vi "Day 2.vi"() -> ()   [LabVIEW 2018]
panel:
  in  "Boolean 2":bool
  in  "Boolean":bool
  in  "Ring":u16(ring)
  in  "Enum":enum16{""}(ring)
  out "x*y":i32
  out "Numeric 2":i32
  out "output cluster 2":cluster{"Numeric 9":dbl, "String":string}
  in  "Cluster 2":cluster{"Numeric 9":dbl, "String":string}
  out "output cluster":T1
  in  "Cluster":T1
  out "x+y":dbl[](array[numeric])
  in  "Array 3":dbl[](array[numeric])
  out "subarray":dbl[][](array[numeric])
  out "min index(es)":i32[](array[numeric])
  out "min value":dbl
  out "max value 2":dbl
  out "max index(es)":i32[](array[numeric])
  in  "max value":dbl
  out "element":dbl
  out "array w/ subset deleted":dbl[](array[numeric])
  out "deleted portion":dbl[](array[numeric])
  out "Array 2":dbl[](array[numeric])
  out "size(s)":i32[](array[numeric])
  out "initialized array":i32[][][](array[numeric])
  out "Array":dbl[][][][][][][][](array[numeric])
  out "Numeric 8":dbl
  out "Numeric 7":dbl
  in  "stop 2":bool
  out "Numeric 6":dbl
  out "Numeric 5":dbl
  out "Numeric 4":dbl
  out "Numeric 3":dbl
  in  "Numeric":i32
  in  "stop":bool
  out "Waveform Chart":dbl(graph)
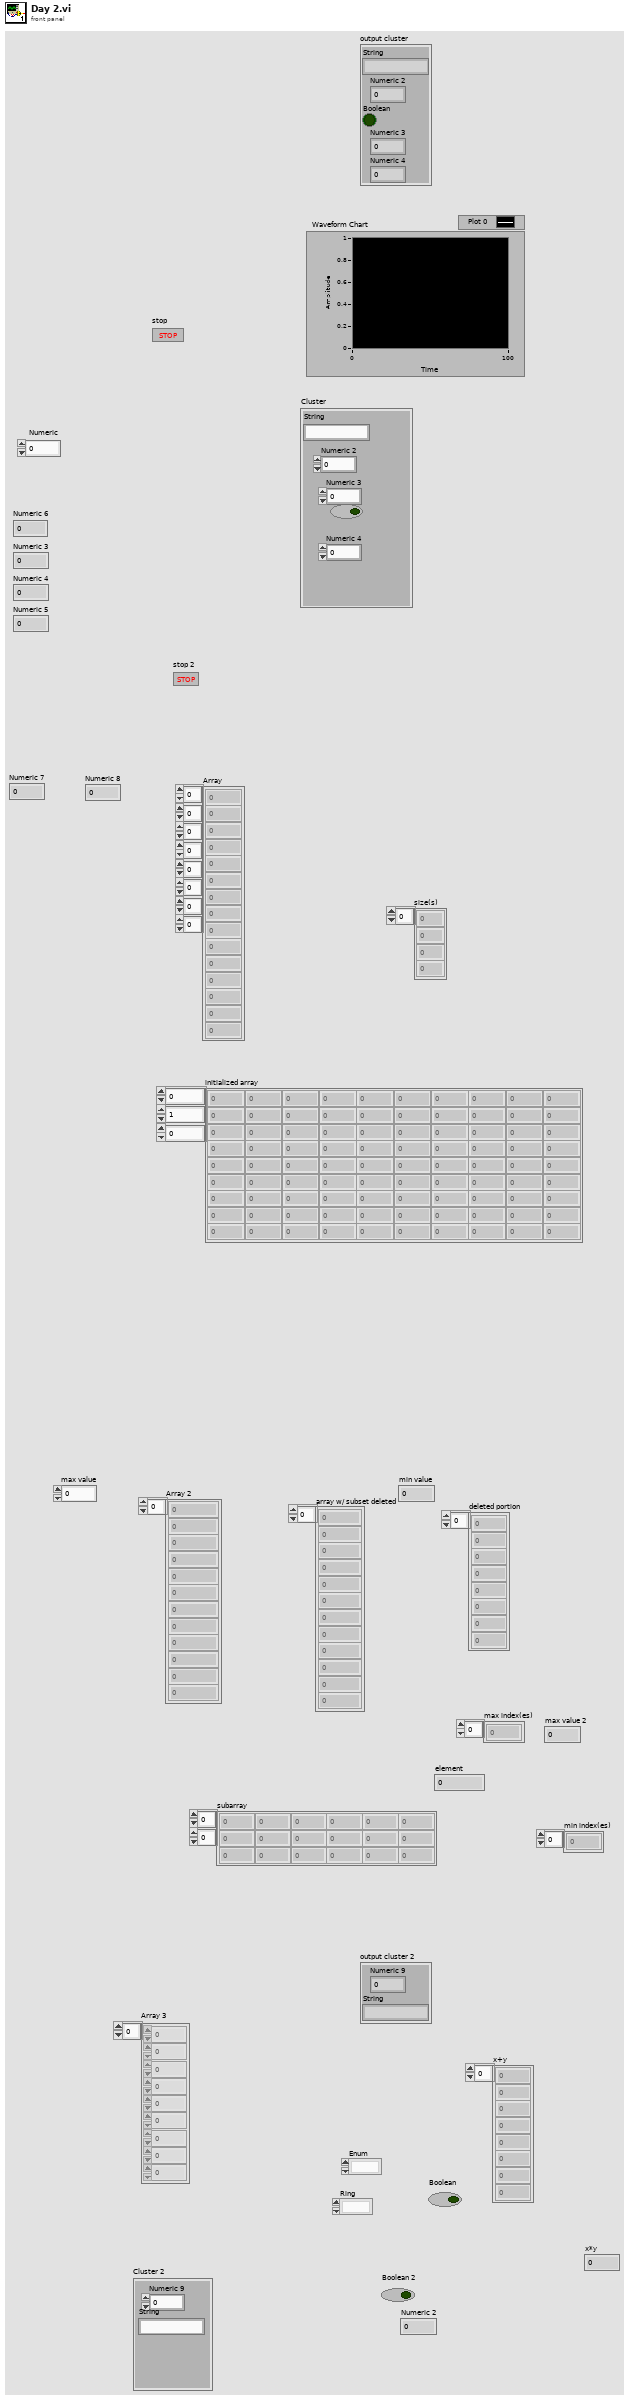
[diagram p1: front panel]
types:
  T1 = cluster{"String":string, "Numeric 2":i32, "Boolean":bool, "Numeric 3":i32, "Numeric 4":i32}
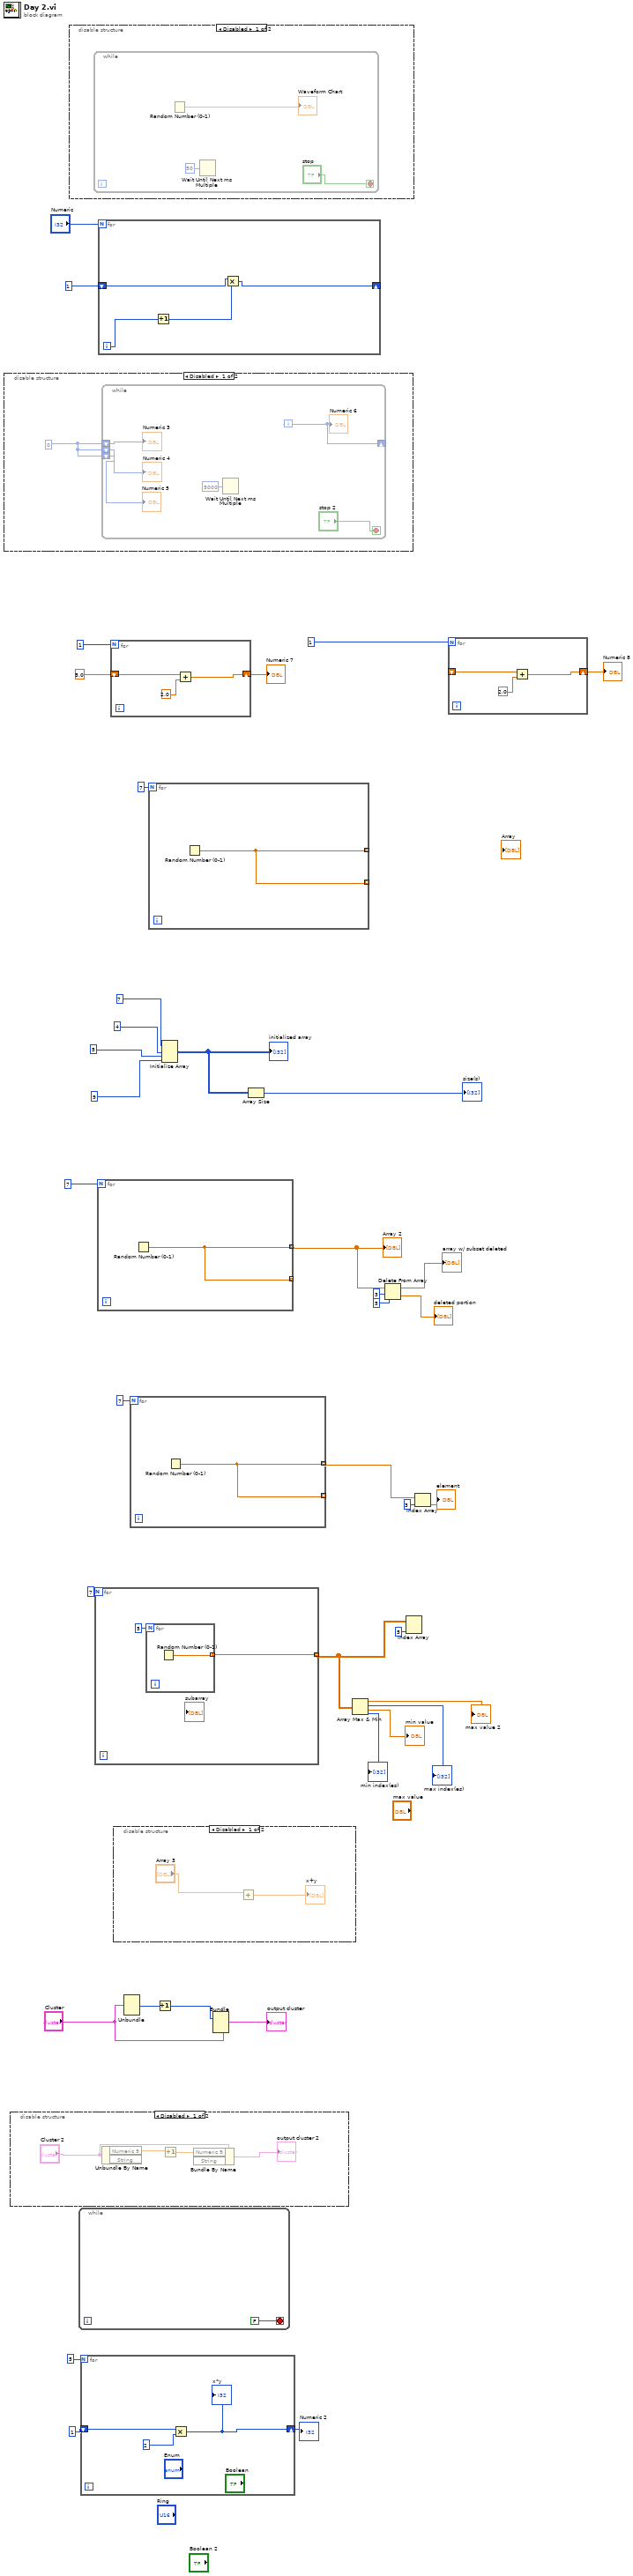
[diagram p0: block diagram]
diagram:
  n1 = disable-structure shown="Disabled" {
    frame Disabled {
      w39 = 0
      n2 = while {
        shift-right: [w42] -> _
        shift-left: w39 -> [w45]
        shift-left: w39 -> [w44]
        shift-left: w39 -> [w43]
        i -> [w42]
        stop <- "stop 2" stop-if-true
        n3 = Wait Until Next ms Multiple(millisecond multiple=u32 5000) -> ()  [unwired: 1 out]
        "Numeric 3" <- w45
        "Numeric 4" <- w44
        "Numeric 5" <- w43
        "Numeric 6" <- w42
      }
    }
    frame Enabled {
    }
  }
  n4 = disable-structure shown="Disabled" {
    frame Disabled {
      n5 = Unbundle By Name("Cluster 2") -> ("Numeric 9"=w49:dbl)  [unwired: 1 out]
      n6 = Increment(x=w49) -> (x+1=w48:dbl)
      n7 = Bundle By Name(cluster="Cluster 2", "Numeric 9"=w48) -> (→"output cluster 2":cluster{"Numeric 9":dbl, "String":string})  [unwired: 1 in]
    }
    frame Enabled {
    }
  }
  n8 = disable-structure shown="Disabled" {
    frame Disabled {
      n9 = while {
        stop <- "stop" stop-if-true
        n10 = Random Number (0-1)() -> (number: 0 to 1=→"Waveform Chart":dbl)
        n11 = Wait Until Next ms Multiple(millisecond multiple=u32 50 ("milliseconds to wait")) -> ()  [unwired: 1 out]
      }
    }
    frame Enabled {
    }
  }
  n12 = while {
    stop <- FALSE stop-if-true
  }
  n13 = for {
    N: 5 -> [_]
    shift-right: [w55] -> w3
    shift-left: 1 -> [w56]
    n14 = Multiply(x=w56, y=2) -> (x*y=w55:i32)
    "x*y" <- w55
  }
  "Numeric 2" <- w3
  n15 = for {
    N: 7 -> [_]
    tunnel: [w58] -> w13 mode=indexing
    n16 = for {
      N: 5 -> [_]
      tunnel: [w59] -> w58 mode=indexing
      n17 = Random Number (0-1)() -> (number: 0 to 1=w59:dbl)
    }
  }
  n18 = for {
    N: 7 -> [_]
    tunnel: [w60] -> w23 mode=indexing
    tunnel: [w60] -> _ mode=indexing
    n19 = Random Number (0-1)() -> (number: 0 to 1=w60:dbl)
  }
  "Array 2" <- w23
  n20 = for {
    N: "Numeric" -> [_]
    shift-right: [w62] -> _
    shift-left: 1 -> [w64]
    i -> [w61]
    n21 = Increment(x=w61) -> (x+1=w63:i32)
    n22 = Multiply(x=w64, y=w63) -> (x*y=w62:i32)
  }
  n23 = for {
    N: 1 -> [_]
    shift-right: [w66] -> w35
    shift-left: 5.0 -> [w67]
    n24 = Add(x=w67, y=2.0) -> (x+y=w66:dbl)
  }
  "Numeric 7" <- w35
  n25 = disable-structure shown="Disabled" {
    frame Disabled {
      n26 = Add(x="Array 3") -> (x+y=→"x+y":dbl[])  [unwired: 1 in]
    }
    frame Enabled {
    }
  }
  n27 = Unbundle("Cluster") -> ("Numeric 2"=w7:i32)  [unwired: 4 out]
  n28 = for {
    N: 7 -> [_]
    tunnel: [w70] -> w17 mode=indexing
    tunnel: [w70] -> _ mode=indexing
    n29 = Random Number (0-1)() -> (number: 0 to 1=w70:dbl)
  }
  n30 = for {
    N: 7 -> [_]
    tunnel: [w71] -> _ mode=indexing
    tunnel: [w71] -> _ mode=indexing
    n31 = Random Number (0-1)() -> (number: 0 to 1=w71:dbl)
  }
  n32 = Increment(x=w7) -> (x+1=w5:i32)
  n33 = Initialize Array(7 ("dimension size"), 4 ("dimension size"), 5 ("dimension size"), 9 ("dimension size")) -> (w26:i32[][][])
  "initialized array" <- w26
  n34 = Bundle(cluster="Cluster", "Numeric 2"=w5) -> (→"output cluster":T1)  [unwired: 4 in]
  n35 = Array Size(array=w26) -> (size(s)=→"size(s)":i32[])
  n36 = Array Max & Min(array=w13) -> (max value=→"max value 2":dbl, max index (indices)=→"max index(es)":i32[], min value=→"min value":dbl, min index (indices)=→"min index(es)":i32[])
  n37 = Delete From Array(array=w23, length=3, index=5) -> (deleted portion=→"deleted portion":dbl[], array with subset deleted=→"array w/ subset deleted":dbl[])
  n38 = Index Array(array=w13, index (col)=5 ("disabled index (col)")) -> ()  [unwired: 1 in, 1 out]
  n39 = Index Array(array=w17, index=3) -> (element=→"element":dbl)
  n40 = for {
    N: 1 -> [_]
    shift-right: [w73] -> w33
    shift-left: _ -> [w74]
    n41 = Add(x=w74, y=2.0) -> (x+y=w73:dbl)
  }
  "Numeric 8" <- w33
